vi "USRP_singlecarrierTDMUSRP1.vi"() -> ()   [LabVIEW 2021]
uses:
  <vilib>/addons/Modulation/Analog/controls/Complex Data Waveform.ctl
  system stop.vi
  <vilib>/measure/matone.llb/Extract Single Tone Information 1 Chan (CDB).vi
  <instrlib>/niUSRP/niUSRP Fetch Rx Data (CDB Cluster).vi
  <instrlib>/niUSRP/niUSRP Write Tx Data (CDB Cluster).vi
  <vilib>/addons/Modulation/niAMT.lvlib
  <vilib>/measure/NI_MAPro.lvlib
panel:
  in  "Tab Control":T1(tab)
  in  "IQ rate Tx":dbl=400000.0 format="%#_6p"
  in  "Tx Gain":dbl format="%#_6f"
  in  "Tx IP":refnum<k15>="192.168.10.2"
  out "coerced IQ rate Tx":dbl=100000.0 format="%#_6p"
  out "coerced carrier frequency Tx":dbl=100000.0 format="%#_6p"
  in  "Rx IP":refnum<k15>="192.168.10.2"
  in  "Rx gain":dbl format="%#_6f"
  in  "Frequency":dbl=10000.0 format="%#_13g"
  in  "Duration":dbl=0.01 format="%#_13g"
  out "coerced IQ rate Rx":dbl=100000.0 format="%#_6p"
  out "coerced carrier frequency Rx":dbl=100000.0 format="%#_6p"
  in  "number of samples":i64=4000
  in  "carrier frequency":dbl=2400000000.0 format="%#_6p"
  in  "Phase in deg":dbl
  out "Waveform Graph":dbl[](graph)
  out "Boolean":bool
  out "detected frequency":dbl format="%.2p"
  out "detected Amplitude in dBm":dbl format="%.2p"
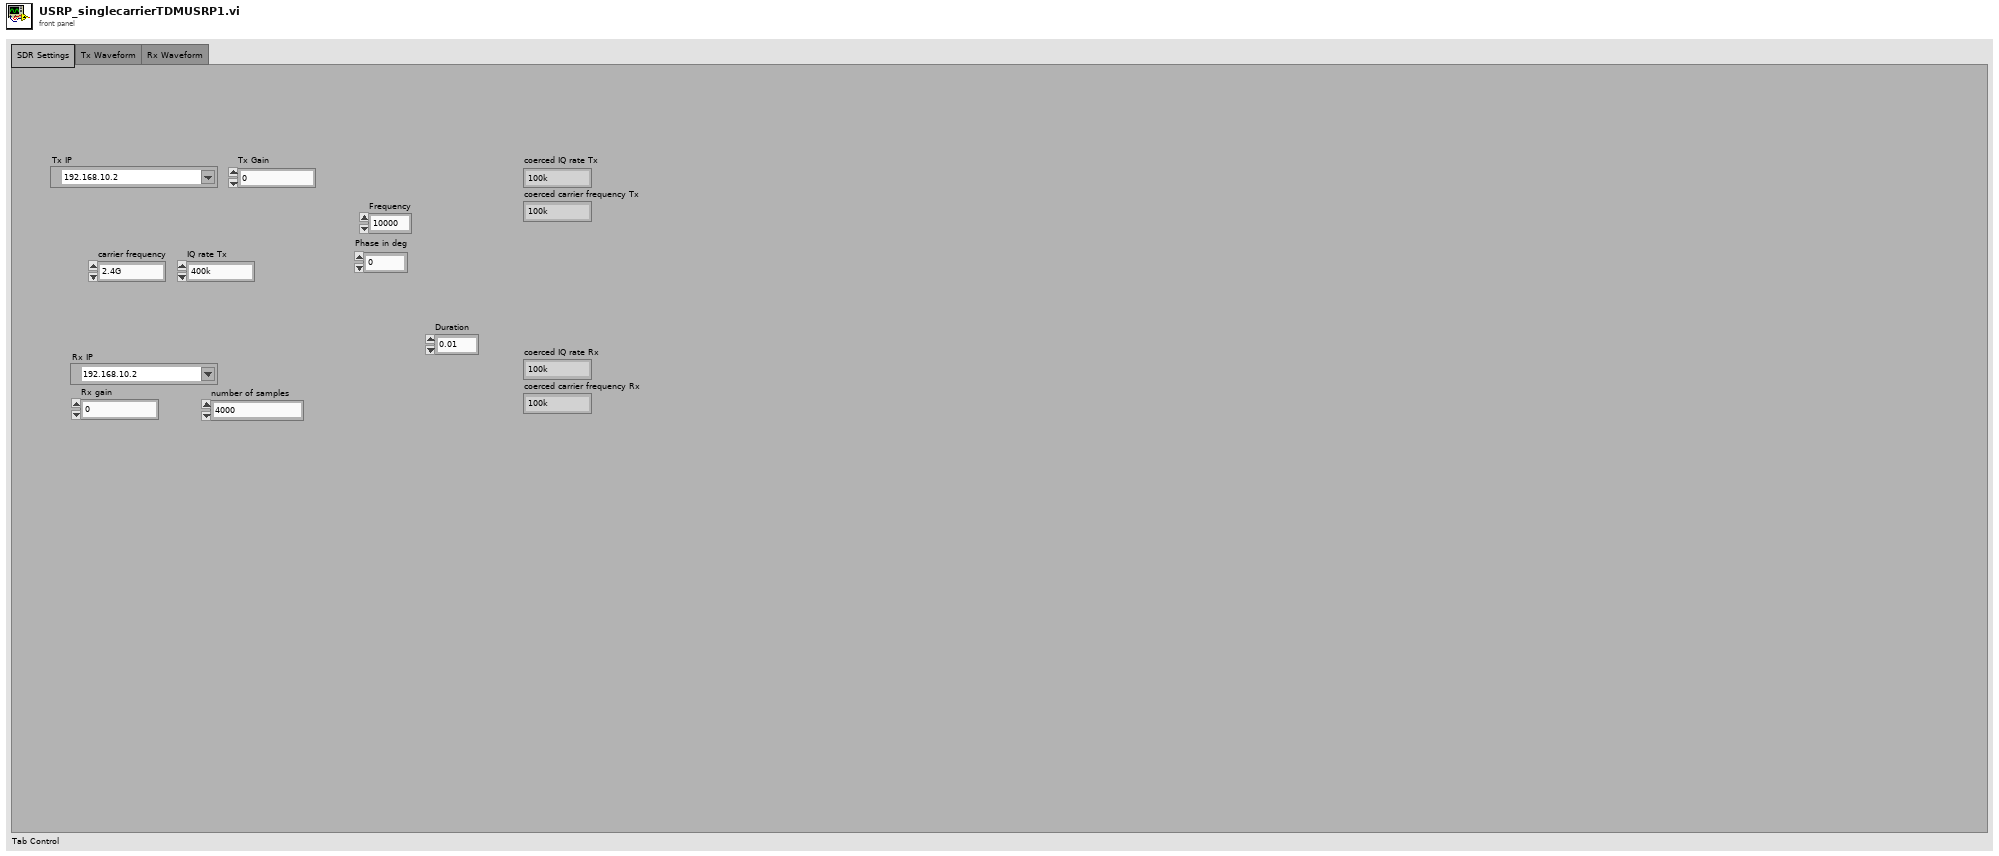
[diagram p1: front panel]
types:
  T1 = enum32{"SDR Settings", "Tx Waveform", "Rx Waveform"}
  T2 = typedef "niAMT.lvlib/Complex Data Waveform.ctl" = cluster{"t0":dbl, "dt":dbl, "Y":cdb[]}
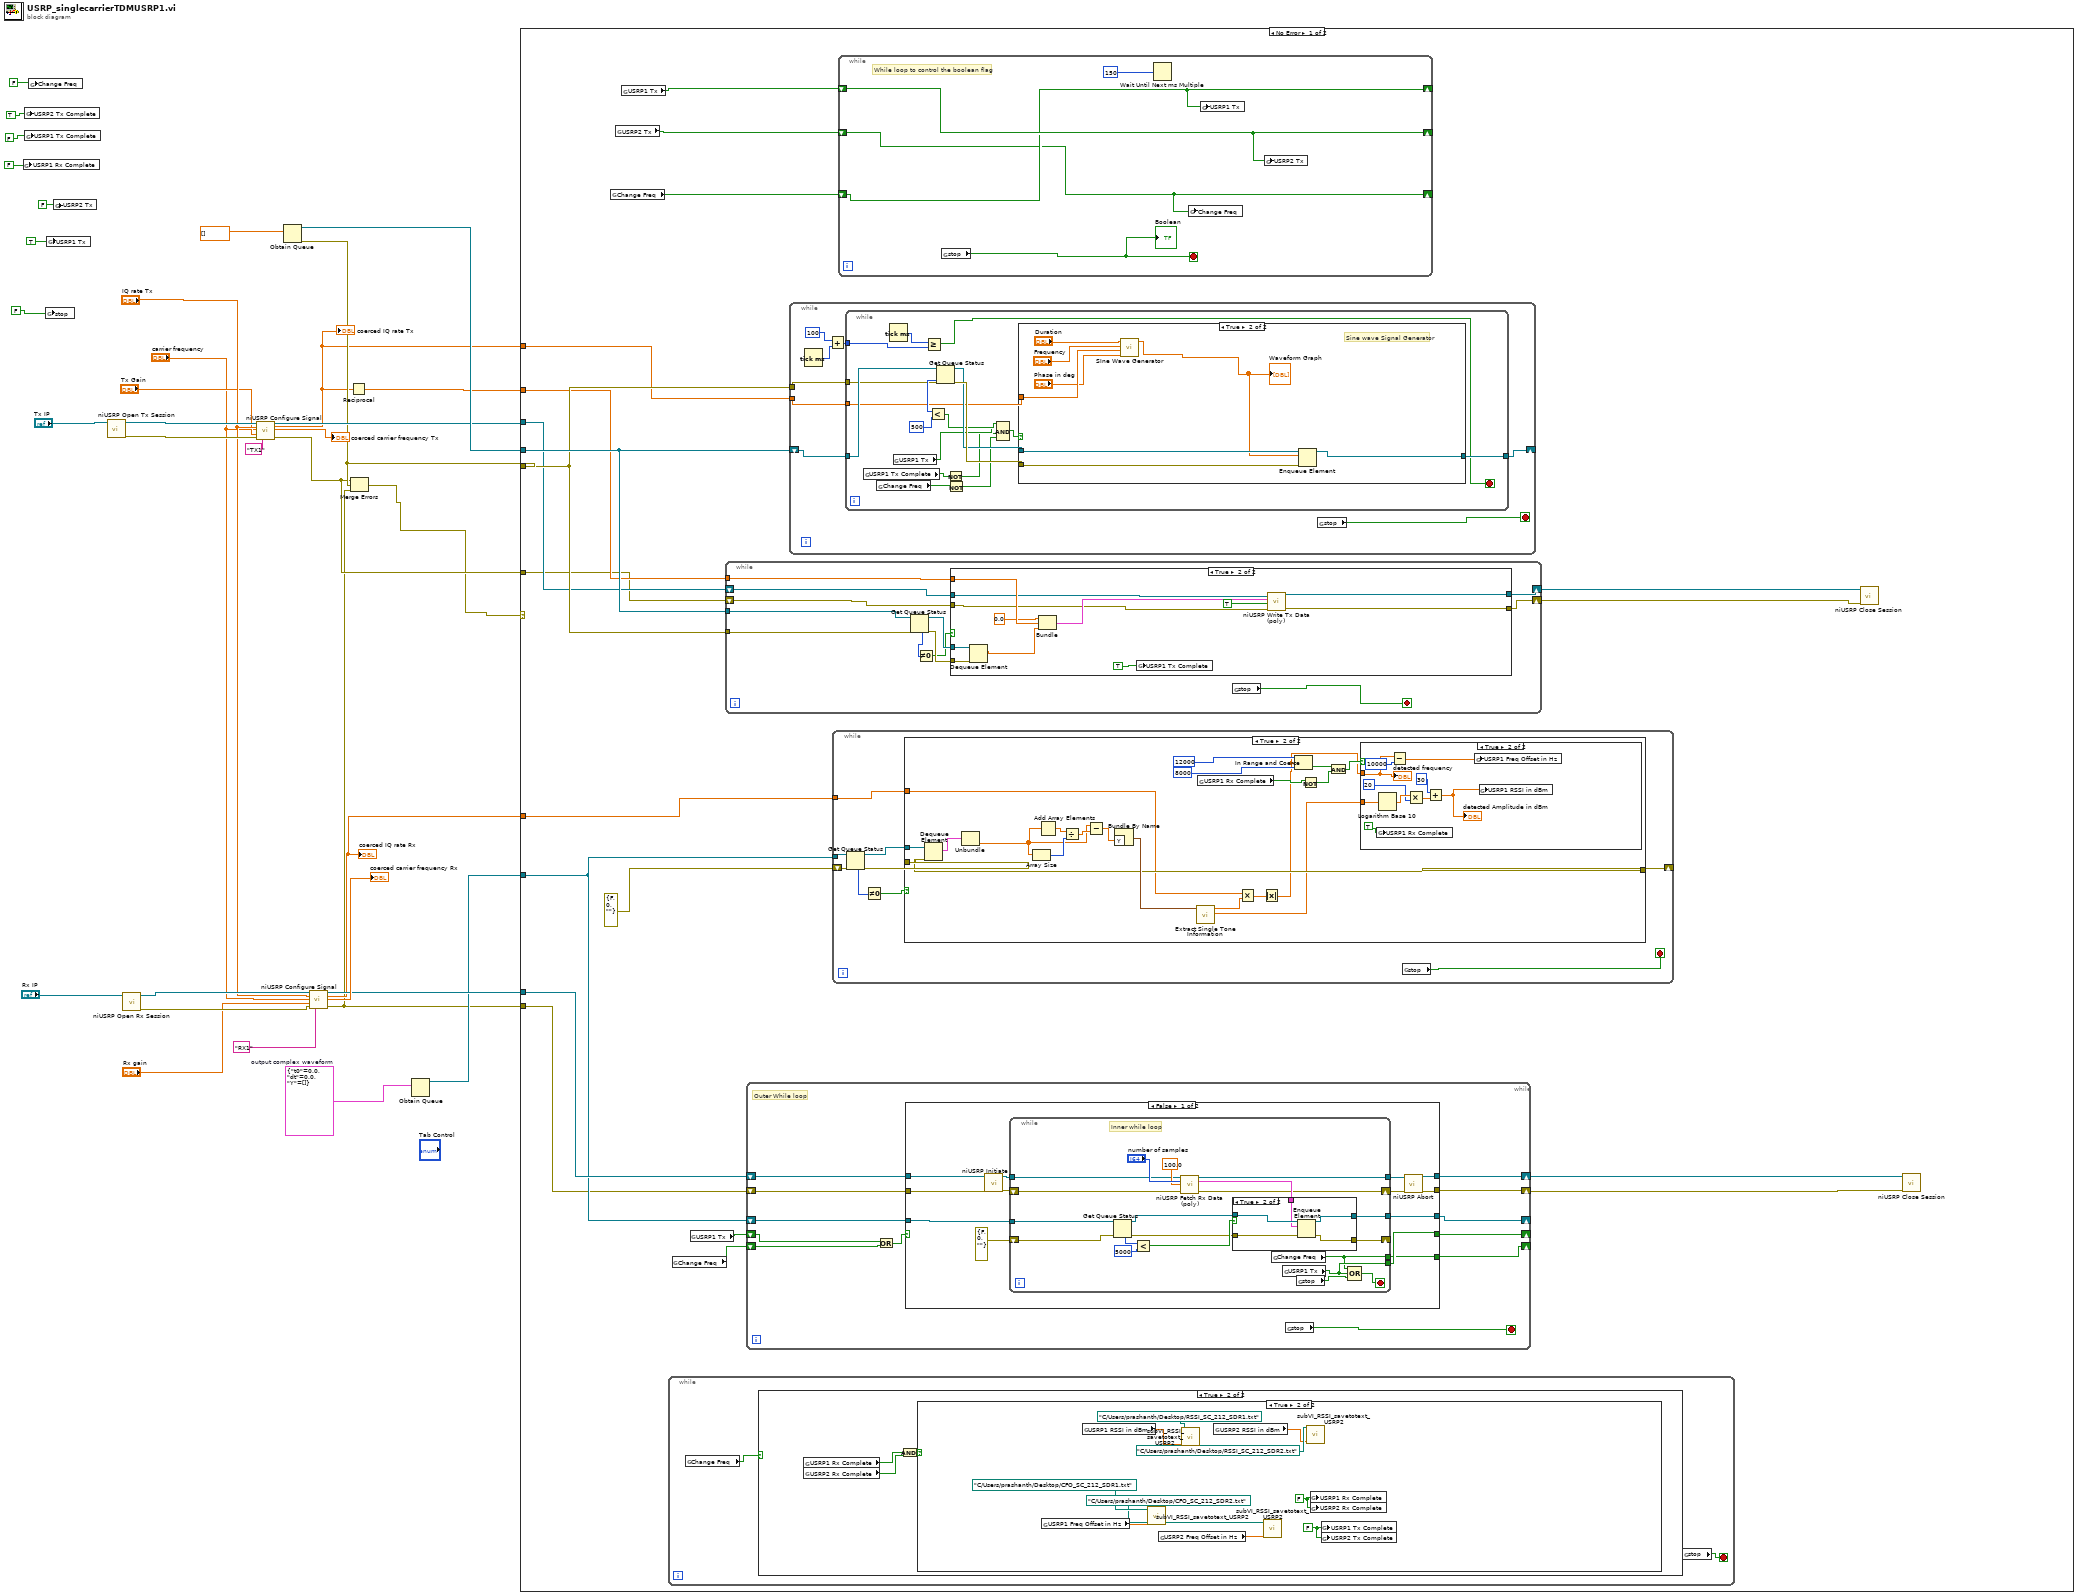
[diagram p0: block diagram]
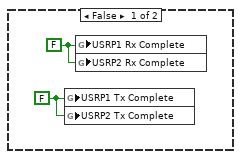
[diagram p3: hidden frame]
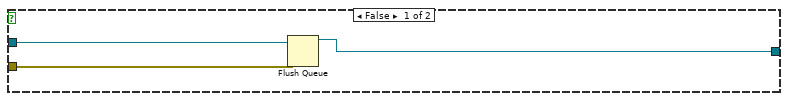
[diagram p4: hidden frame]
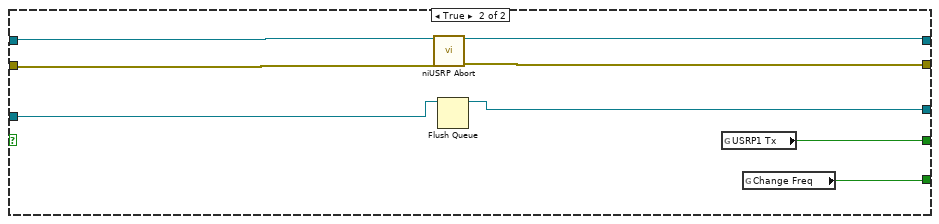
[diagram p6: hidden frame]
diagram:
  w8 = T2 {"t0"=0.0, "dt"=0.0, "Y"=[]}  # output complex waveform
  n1 = global write "system stop.vi" "USRP1 Rx Complete"(FALSE) -> ()
  n2 = global write "system stop.vi" "USRP2 Tx Complete"(TRUE) -> ()
  n3 = global write "system stop.vi" "USRP1 Tx Complete"(FALSE) -> ()
  n4 = global write "system stop.vi" "Change Freq"(FALSE) -> ()
  n5 = global write "system stop.vi" "stop"(FALSE) -> ()
  n6 = global write "system stop.vi" "USRP1 Tx"(TRUE) -> ()
  n7 = global write "system stop.vi" "USRP2 Tx"(FALSE) -> ()
  n8 = call <instrlib>:"niUSRP Open Tx Session.vi"("device names"="Tx IP") -> ("session handle out"=w33:refnum<k15>, "error out"=w32:errorcluster)  [unwired: 13 in]
  n9 = call <instrlib>:"niUSRP Open Rx Session.vi"("device names"="Rx IP") -> ("session handle out"=w30:refnum<k15>, "error out"=w29:errorcluster)  [unwired: 13 in]
  n10 = call <instrlib>:"niUSRP Configure Signal.vi"("session handle"=w33, "IQ rate"="IQ rate Tx", "carrier frequency"="carrier frequency", "gain"="Tx Gain", "error in (no error)"=w32, "active antenna"="TX1") -> ("session handle out"=w15:refnum<k15>, "coerced IQ rate"=w12:dbl, "coerced carrier frequency"=→"coerced carrier frequency Tx":dbl, "error out"=w11:errorcluster)  [unwired: 5 in, 1 out]
  "coerced IQ rate Tx" <- w12
  n11 = Obtain Queue(element data type=dbl[] []) -> (queue out=w16:refnum<queue>, error out=w13:errorcluster)  [unwired: 4 in, 1 out]
  n12 = call <instrlib>:"niUSRP Configure Signal.vi"("session handle"=w30, "IQ rate"="IQ rate Tx", "carrier frequency"="carrier frequency", "gain"="Rx gain", "error in (no error)"=w29, "active antenna"="RX1") -> ("session handle out"=w9:refnum<k15>, "coerced IQ rate"=w6:dbl, "coerced carrier frequency"=→"coerced carrier frequency Rx":dbl, "error out"=w4:errorcluster)  [unwired: 5 in, 1 out]
  "coerced IQ rate Rx" <- w6
  n13 = Reciprocal(x=w12) -> (1/x=w14:dbl)
  n14 = Merge Errors(w11, w13, w4) -> (w2:errorcluster)
  n15 = Obtain Queue(element data type=w8) -> (queue out=w7:refnum<queue>)  [unwired: 4 in, 2 out]
  n16 = case shown="No Error" w2 {
    tunnel: w13 -> [w53 _]
    tunnel: w16 -> [w54 _]
    tunnel: w15 -> [w51 _]
    tunnel: w14 -> [w52 _]
    tunnel: w12 -> [w50 _]
    tunnel: w11 -> [w49 _]
    tunnel: w9 -> [w47 _]
    tunnel: w7 -> [w46 _]
    tunnel: w6 -> [w45 _]
    tunnel: w4 -> [w44 _]
    frame No Error {
      n17 = global read "system stop.vi" "Change Freq"() -> (w36:bool)
      n18 = global read "system stop.vi" "USRP2 Tx"() -> (w41:bool)
      n19 = global read "system stop.vi" "USRP1 Tx"() -> (w42:bool)
      n20 = while {
        stop <- w55 stop-if-true
        n21 = global read "system stop.vi" "Change Freq"() -> (w56:bool)
        n22 = case shown="True" w56 {
          frame False {
          }
          frame True {
            n23 = global read "system stop.vi" "USRP1 Rx Complete"() -> (w59:bool)
            n24 = global read "system stop.vi" "USRP2 Rx Complete"() -> (w58:bool)
            n25 = And(x=w59, y=w58) -> (x .and. y?=w57:bool)
            n26 = case shown="True" w57 {
              frame False {
                w61 = FALSE
                w60 = FALSE
                n27 = global write "system stop.vi" "USRP1 Tx Complete"(w61) -> ()
                n28 = global write "system stop.vi" "USRP2 Tx Complete"(w61) -> ()
                n29 = global write "system stop.vi" "USRP1 Rx Complete"(w60) -> ()
                n30 = global write "system stop.vi" "USRP2 Rx Complete"(w60) -> ()
              }
              frame True {
                w71 = FALSE
                w70 = FALSE
                n31 = global read "system stop.vi" "USRP1 Freq Offset in Hz"() -> (w64:dbl)
                n32 = global read "system stop.vi" "USRP1 RSSI in dBm"() -> (w68:dbl)
                n33 = call "subVI_RSSI_savetotext_USRP2.vi"("RSSI"=w64, "file path (dialog if empty)"=path "C:/Users/prashanth/Desktop/CFO_SC_212_SDR1.txt") -> ()  [unwired: 10 in]
                n34 = global read "system stop.vi" "USRP2 Freq Offset in Hz"() -> (w62:dbl)
                n35 = call "subVI_RSSI_savetotext_USRP2.vi"("RSSI"=w68, "file path (dialog if empty)"=path "C:/Users/prashanth/Desktop/RSSI_SC_212_SDR1.txt") -> ()  [unwired: 10 in]
                n36 = global read "system stop.vi" "USRP2 RSSI in dBm"() -> (w66:dbl)
                n37 = call "subVI_RSSI_savetotext_USRP2.vi"("RSSI"=w62, "file path (dialog if empty)"=path "C:/Users/prashanth/Desktop/CFO_SC_212_SDR2.txt") -> ()  [unwired: 10 in]
                n38 = call "subVI_RSSI_savetotext_USRP2.vi"("RSSI"=w66, "file path (dialog if empty)"=path "C:/Users/prashanth/Desktop/RSSI_SC_212_SDR2.txt") -> ()  [unwired: 10 in]
                n39 = global write "system stop.vi" "USRP1 Rx Complete"(w70) -> ()
                n40 = global write "system stop.vi" "USRP2 Rx Complete"(w70) -> ()
                n41 = global write "system stop.vi" "USRP1 Tx Complete"(w71) -> ()
                n42 = global write "system stop.vi" "USRP2 Tx Complete"(w71) -> ()
              }
            }
          }
        }
        n43 = global read "system stop.vi" "stop"() -> (w55:bool)
      }
      n44 = global read "system stop.vi" "Change Freq"() -> (w35:bool)
      n45 = global read "system stop.vi" "USRP1 Tx"() -> (w43:bool)
      n46 = while {
        tunnel: w54 -> [w226]
        tunnel: w53 -> [w223]
        tunnel: w52 -> [w222]
        shift-right: [w219] -> w38
        shift-left: w51 -> [w216]
        shift-right: [w218] -> w37
        shift-left: w49 -> [w215]
        stop <- w217 stop-if-true
        n47 = Get Queue Status(queue=w226, error in (no error)=w223) -> (queue out=w225:refnum<queue>, error out=w224:errorcluster, # elements in queue=w221:i32)  [unwired: 1 in, 5 out]
        n48 = Not Equal To 0?(x=w221) -> (x != 0?=w220:bool)
        n49 = case shown="True" w220 {
          tunnel: w225 -> [_ w240]
          tunnel: w224 -> [_ w239]
          tunnel: w222 -> [_ w238]
          tunnel: w216 -> [w228 w231]
          tunnel: w215 -> [w227 w230]
          tunnel: [w228 w234] -> w219
          tunnel: [w227 w232] -> w218
          frame False {
          }
          frame True {
            n50 = Dequeue Element(queue=w240, error in (no error)=w239) -> (element=w229:dbl[])  [unwired: 1 in, 3 out]
            n51 = Bundle(0.0, w238, w229) -> (w237:cluster{dbl, dbl, dbl[]})  [unwired: 1 in]
            n52 = global write "system stop.vi" "USRP1 Tx Complete"(TRUE) -> ()
            n53 = call-poly <instrlib>:"niUSRP Write Tx Data (poly).vi"("session handle"=w231, "data"=w237, "end of data?"=TRUE, "error in (no error)"=w230) -> ("session handle out"=w234:refnum<k15>, "error out"=w232:errorcluster)  [unwired: 10 in]
          }
        }
        n54 = global read "system stop.vi" "stop"() -> (w217:bool)
      }
      n55 = while {
        shift-right: [w122] -> _
        shift-left: w43 -> [w120]
        shift-right: [w124] -> w40
        shift-left: w47 -> [w116]
        shift-right: [w123] -> w39
        shift-left: w44 -> [w115]
        shift-right: [w118] -> _
        shift-left: w35 -> [w117]
        shift-right: [w114] -> _
        shift-left: w46 -> [w125]
        stop <- w121 stop-if-true
        # "Outer While loop"
        n56 = Or(x=w120, y=w117) -> (x .or. y?=w119:bool)
        n57 = case shown="False" w119 {
          tunnel: w116 -> [w128 w172]
          tunnel: w125 -> [w138 w168]
          tunnel: w115 -> [w127 w170]
          tunnel: [w132 w171] -> w124
          tunnel: [w131 w169] -> w123
          tunnel: [w136 w173] -> w122
          tunnel: [w129 w167] -> w118
          tunnel: [w126 w166] -> w114
          frame False {
            n58 = call <instrlib>:"niUSRP Initiate.vi"("session handle"=w128, "error in (no error)"=w127) -> ("session handle out"=w135:refnum<k15>, "error out"=w134:errorcluster)  [unwired: 12 in]
            n59 = while {
              tunnel: w138 -> [w158]
              shift-right: [w142] -> w130
              shift-left: w134 -> [w144]
              shift-right: [w157] -> _
              shift-left: errorcluster {"status"=FALSE, "code"=0, "source"=""} ("error in (no error)") -> [w156]
              tunnel: [w141] -> w136
              tunnel: w135 -> [w145]
              tunnel: [w143] -> w133
              tunnel: [w140] -> w129
              tunnel: [w139] -> w126
              stop <- w148 stop-if-true
              # "Inner while loop"
              n60 = Get Queue Status(queue=w158, error in (no error)=w156) -> (queue out=w151:refnum<queue>, error out=w152:errorcluster, # elements in queue=w155:i32)  [unwired: 1 in, 5 out]
              n61 = Less?(x=w155, y=5000) -> (x < y?=w153:bool)
              n62 = call-poly <instrlib>:"niUSRP Fetch Rx Data (poly).vi"("session handle"=w145, "number of samples"="number of samples", "timeout"=100.0, "error in (no error)"=w144) -> ("session handle out"=w143:refnum<k15>, "data"=w149:cluster{"t0":dbl, "dt":dbl, "Y":cdb[]}, "error out"=w142:errorcluster)  [unwired: 8 in, 1 out]
              n63 = case shown="True" w153 {
                tunnel: w152 -> [w160 w165]
                tunnel: w151 -> [w159 w164]
                tunnel: w149 -> [_ w163]
                tunnel: [w160 w162] -> w157
                tunnel: [w159 w161] -> w139
                frame False {
                }
                frame True {
                  n64 = Enqueue Element(queue=w164, element=w163, error in (no error)=w165) -> (queue out=w161:refnum<queue>, error out=w162:errorcluster)  [unwired: 1 in, 1 out]
                }
              }
              n65 = global read "system stop.vi" "Change Freq"() -> (w140:bool)
              n66 = global read "system stop.vi" "USRP1 Tx"() -> (w141:bool)
              n67 = global read "system stop.vi" "stop"() -> (w147:bool)
              n68 = Compound Arithmetic op=OR(w140, w141, w147) -> (w148:bool)
            }
            n69 = call <instrlib>:"niUSRP Abort.vi"("session handle"=w133, "error in (no error)"=w130) -> ("session handle out"=w132:refnum<k15>, "error out"=w131:errorcluster)  [unwired: 12 in]
          }
          frame True {
            n70 = call <instrlib>:"niUSRP Abort.vi"("session handle"=w172, "error in (no error)"=w170) -> ("session handle out"=w171:refnum<k15>, "error out"=w169:errorcluster)  [unwired: 12 in]
            n71 = Flush Queue(queue=w168) -> (queue out=w166:refnum<queue>)  [unwired: 1 in, 2 out]
            n72 = global read "system stop.vi" "USRP1 Tx"() -> (w173:bool)
            n73 = global read "system stop.vi" "Change Freq"() -> (w167:bool)
          }
        }
        n74 = global read "system stop.vi" "stop"() -> (w121:bool)
      }
      n75 = while {
        tunnel: w53 -> [w83]
        tunnel: w50 -> [w82]
        shift-right: [w77] -> _
        shift-left: w54 -> [w84]
        stop <- w78 stop-if-true
        n76 = Tick Count (ms)() -> (millisecond timer value=w80:u32)
        n77 = Add(x=100, y=w80) -> (x+y=w79:u32)
        n78 = while {
          tunnel: w83 -> [w97]
          tunnel: w82 -> [w96]
          tunnel: w79 -> [w91]
          tunnel: w84 -> [w98]
          tunnel: [w89] -> w77
          stop <- w86 stop-if-true
          n79 = global read "system stop.vi" "USRP1 Tx Complete"() -> (w88:bool)
          n80 = global read "system stop.vi" "Change Freq"() -> (w87:bool)
          n81 = Tick Count (ms)() -> (millisecond timer value=w92:u32)
          n82 = global read "system stop.vi" "USRP1 Tx"() -> (w94:bool)
          n83 = Greater Or Equal?(x=w92, y=w91) -> (x >= y?=w86:bool)
          n84 = Get Queue Status(queue=w98, error in (no error)=w97) -> (queue out=w99:refnum<queue>, error out=w100:errorcluster, # elements in queue=w102:i32)  [unwired: 1 in, 5 out]
          n85 = Less?(x=w102, y=500) -> (x < y?=w95:bool)
          n86 = Not(x=w88) -> (.not. x?=w90:bool)
          n87 = Not(x=w87) -> (.not. x?=w85:bool)
          n88 = Compound Arithmetic op=AND(w95, w94, w90, w85) -> (w93:bool)
          n89 = case shown="True" w93 {
            tunnel: w100 -> [w104 w113]
            tunnel: w99 -> [w105 w112]
            tunnel: w96 -> [_ w108]
            tunnel: [w103 w110] -> w89
            frame False {
              n90 = Flush Queue(queue=w105, error in (no error)=w104) -> (queue out=w103:refnum<queue>)  [unwired: 2 out]
            }
            frame True {
              # "Sine wave Signal Generator"
              n91 = call "SIne Wave Generator.vi"("Phase in deg"="Phase in deg", "Sampling rate"=w108, "Frequency"="Frequency", "Duration"="Duration") -> ("Array"=w106:dbl[])  [unwired: 6 in, 1 out]
              "Waveform Graph" <- w106
              n92 = Enqueue Element(queue=w112, element=w106, error in (no error)=w113) -> (queue out=w110:refnum<queue>)  [unwired: 1 in, 2 out]
            }
          }
        }
        n93 = global read "system stop.vi" "stop"() -> (w78:bool)
      }
      n94 = while {
        tunnel: w46 -> [w179]
        shift-right: [w176] -> _
        shift-left: errorcluster {"status"=FALSE, "code"=0, "source"=""} ("error in (no error)") -> [w178]
        tunnel: w45 -> [w175]
        stop <- w174 stop-if-true
        n95 = Get Queue Status(queue=w179, error in (no error)=w178) -> (queue out=w181:refnum<queue>, error out=w180:errorcluster, # elements in queue=w182:i32)  [unwired: 1 in, 5 out]
        n96 = Not Equal To 0?(x=w182) -> (x != 0?=w177:bool)
        n97 = case shown="True" w177 {
          tunnel: w181 -> [_ w204]
          tunnel: w180 -> [w183 w203]
          tunnel: [w183 w190] -> w176
          tunnel: w175 -> [_ w186]
          frame False {
          }
          frame True {
            n98 = Dequeue Element(queue=w204, error in (no error)=w203) -> (element=w202:T2, error out=w190:errorcluster)  [unwired: 1 in, 2 out]
            n99 = Unbundle(w202) -> ("Y"=w189:cdb[])  [unwired: 2 out]
            n100 = Array Size(array=w189) -> (size(s)=w200:i32)
            n101 = Add Array Elements(numeric array=w189) -> (sum=w201:cdb)
            n102 = Divide(x=w201, y=w200) -> (x/y=w199:cdb)
            n103 = Subtract(x=w189, y=w199) -> (x-y=w198:cdb[])
            n104 = Bundle By Name("Y"=w198) -> (w191:waveform(cdb))  [unwired: 1 in]
            n105 = call-poly <vilib>:"Extract Single Tone Information.vi"("time signal in"=w191) -> ("detected amplitude"=w188:dbl, "detected frequency"=w187:dbl)  [unwired: 5 in, 4 out]
            n106 = global read "system stop.vi" "USRP1 Rx Complete"() -> (w193:bool)
            n107 = Multiply(x=w186, y=w187) -> (x*y=w185:dbl)
            n108 = Absolute Value(x=w185) -> (abs(x)=w184:dbl)
            n109 = In Range and Coerce(upper limit=12000, x=w184, lower limit=8000) -> (In Range?=w194:bool)  [unwired: 1 out]
            n110 = Not(x=w193) -> (.not. x?=w192:bool)
            n111 = And(x=w194, y=w192) -> (x .and. y?=w195:bool)
            n112 = case shown="True" w195 {
              tunnel: w184 -> [_ w208]
              tunnel: w188 -> [_ w205]
              frame False {
              }
              frame True {
                n113 = global write "system stop.vi" "USRP1 Rx Complete"(TRUE) -> ()
                n114 = Logarithm Base 10(1:w205) -> (0:w214:dbl)
                n115 = Subtract(x=w208, y=10000) -> (x-y=w206:dbl)
                n116 = Multiply(x=w214, y=20) -> (x*y=w211:dbl)
                n117 = Add(x=30, y=w211) -> (x+y=w209:dbl)
                "detected Amplitude in dBm" <- w209
                n118 = global write "system stop.vi" "USRP1 Freq Offset in Hz"(w206) -> ()
                n119 = global write "system stop.vi" "USRP1 RSSI in dBm"(w209) -> ()
                "detected frequency" <- w208
              }
            }
          }
        }
        n120 = global read "system stop.vi" "stop"() -> (w174:bool)
      }
      n121 = while {
        shift-right: [w73] -> _
        shift-left: w42 -> [w75]
        shift-right: [w75] -> _
        shift-left: w41 -> [w72]
        shift-right: [w72] -> _
        shift-left: w36 -> [w73]
        stop <- w74 stop-if-true
        # "While loop to control the boolean flag"
        n122 = global read "system stop.vi" "stop"() -> (w74:bool)
        "Boolean" <- w74
        n123 = Wait Until Next ms Multiple(millisecond multiple=150) -> ()  [unwired: 1 out]
        n124 = global write "system stop.vi" "Change Freq"(w72) -> ()
        n125 = global write "system stop.vi" "USRP1 Tx"(w73) -> ()
        n126 = global write "system stop.vi" "USRP2 Tx"(w75) -> ()
      }
      n127 = call <instrlib>:"niUSRP Close Session.vi"("session handle"=w38, "error in (no error)"=w37) -> ()  [unwired: 13 in, 1 out]
      n128 = call <instrlib>:"niUSRP Close Session.vi"("session handle"=w40, "error in (no error)"=w39) -> ()  [unwired: 13 in, 1 out]
    }
    frame Error {
    }
  }
